vi "PicoScope4000ExampleStreaming.vi"() -> ()   [LabVIEW 2012]
doc: "This example demonstrates how to use the PicoScope Labview library to stream data from a PicoScope 4000 Series Device"
uses:
  PicoScope4000Lib/PicoScope4000AnalogChannelSettingsIEPE.ctl
  PicoScope4000Lib/PicoScope4000Buffer and Transfer Settings.ctl
panel:
  in  "Channel B Settings":T1={"Enabled"=FALSE, "Range"=6, "Bandwidth Limit"=0, "Coupling"=1} {"Coupling" items=["AC", "DC", "IEPE"]; "Bandwidth Limit" items=["Off", "200kHz"]; "Range" items=["10 mV", "20 mV", "50 mV", "100 mV", "200 mV", "500 mV", "1 V", "2 V", "5 V", "10 V", "20 V", "50 V ", "100 V"]}
  out "Unit Info":T2
  in  "Channel A Settings":T1={"Enabled"=TRUE, "Range"=6, "Bandwidth Limit"=0, "Coupling"=1} {"Coupling" items=["AC", "DC", "IEPE"]; "Bandwidth Limit" items=["Off", "200kHz"]; "Range" items=["10 mV", "20 mV", "50 mV", "100 mV", "200 mV", "500 mV", "1 V", "2 V", "5 V", "10 V", "20 V", "50 V ", "100 V"]}
  out "Analog Channels":cluster{i32, dbl, "Data (Volts)":dbl[]}[](graph)=[{0, 8e-09, "Data (Volts)"=[]}, {0, 8e-09, "Data (Volts)"=[]}, {0, 8e-09, "Data (Volts)"=[]}, {0, 8e-09, "Data (Volts)"=[]}, {0, 8e-09, "Data (Volts)"=[]}, {0, 8e-09, "Data (Volts)"=[]}, {0, 8e-09, "Data (Volts)"=[]}, {0, 8e-09, "Data (Volts)"=[]}]
  out "Raw Sample Interval (sec)":dbl format="%#.5p"
  out "Max ADC value":i16
  out "Chunk time(ms)":u32
  out "Elapsed time":dbl
  in  "Data file":path=path "PicoScope4000aExampleStreaming ChA Data"
  out "size(s)":i32
  out "Queue depth":i32(graph)
  out "queue depth":i32
  in  "Buffer and Transfer Settings":T3={"startIndex"=0, "Samples"=1000000, "Down Sample Ratio"=1, "Down-Sample Mode"=0} {"Down-Sample Mode" items=["None", "Aggregate", "Average"]; "Down Sample Ratio" step=1; "Samples" format="%_6p"}
  out "TriggeredAt (In Buffer)":u32 format="%#.6p"
  out "TriggeredAt (Total samples)":u32 format="%#.6p"
  in  "Acquisition Settings":T4={"Auto Stop"=TRUE, "Desired Sample Interval"=1, "Pre-trigger Samples"=0, "Post-trigger Samples"=1000000, "Down-Sample Ratio"=1, "Down-Sample Mode"=0, "Time Units"=3} {"Time Units" items=["Nanoseconds (ns)"=2, "Microseconds (us)"=3, "Milliseconds (ms)"=4, "Seconds (s)"=5]; "Down-Sample Mode" items=["None"=0, "Aggregate"=1, "Decimate"=2, "Average"=4]; "Post-trigger Samples" format="%#.6p"; "Pre-trigger Samples" format="%#_6p"}
  out "Triggered":bool
  out "DownSample Interval (sec)":dbl format="%#.5p"
  out "Total Samples":u32 format="%#.6p"
  out "Auto Stopped":bool
  in  "Serial Number":string
  in  "Open Using Serial Number":bool
  out "Number of Samples per Capture":u32 format="%#.6p"
  in  "Apply  Settings":bool
  in  "stop":bool
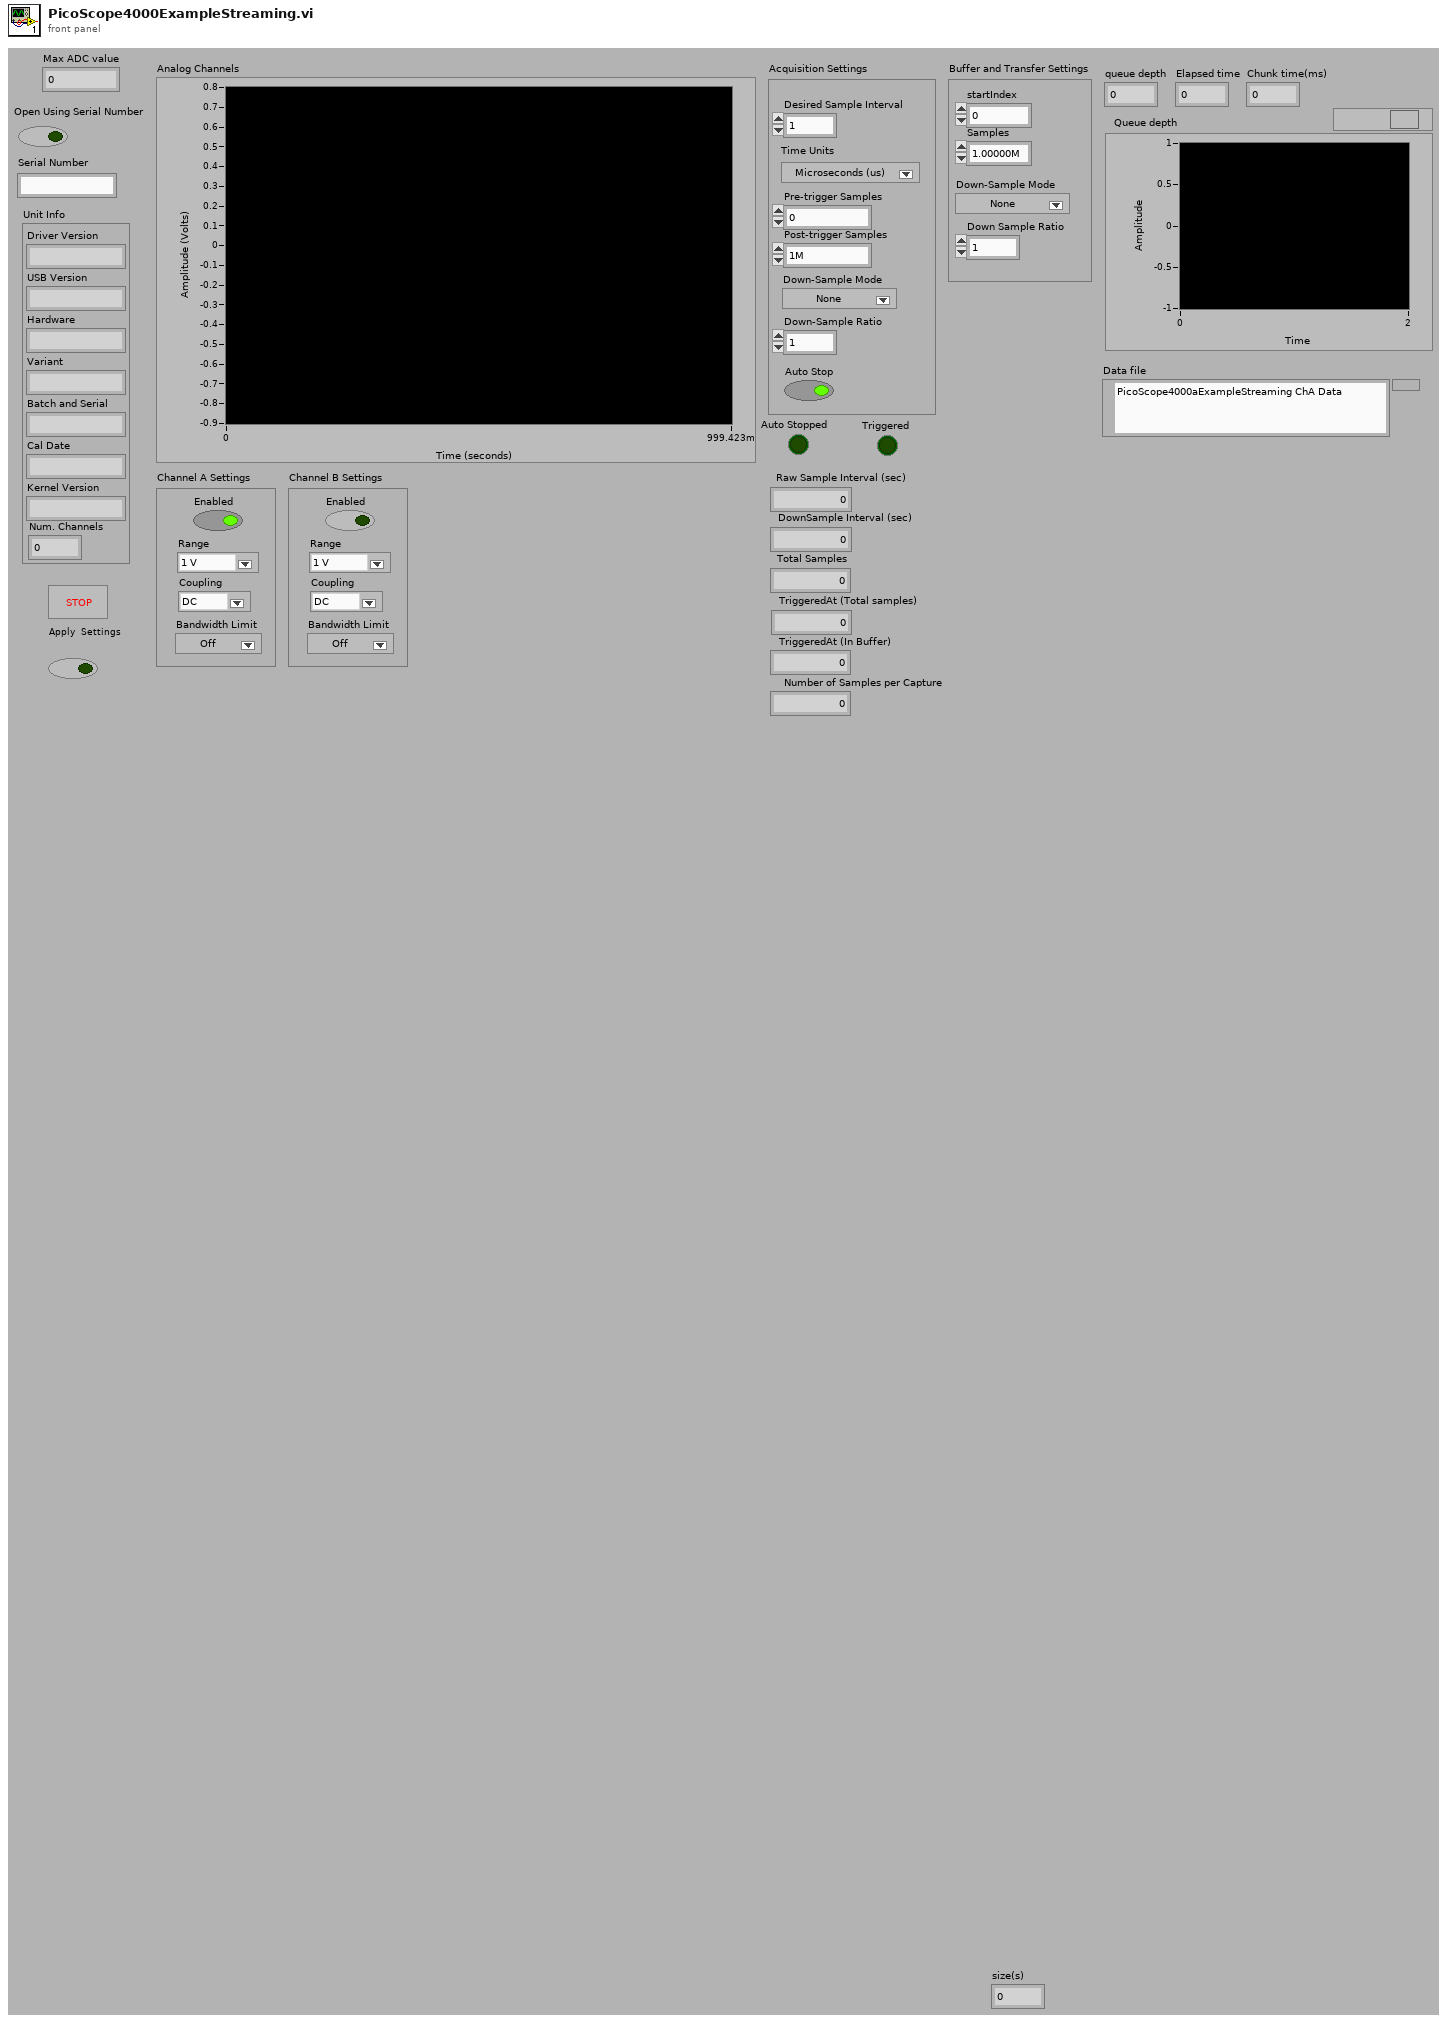
[diagram p1: front panel]
types:
  T1 = typedef "PicoScope4000AnalogChannelSettingsIEPE.ctl" = cluster{"Enabled":bool, "Range":u16, "Bandwidth Limit":i16, "Coupling":u16}
  T2 = cluster{"Driver Version":string, "USB Version":string, "Hardware":string, "Variant":string, "Batch and Serial":string, "Cal Date":string, "Kernel Version":string, "Num. Channels":i16}
  T3 = typedef "PicoScope4000Buffer and Transfer Settings.ctl" = cluster{"startIndex":u64, "Samples":u64, "Down Sample Ratio":u64, "Down-Sample Mode":u32}
  T4 = cluster{"Auto Stop":bool, "Desired Sample Interval":u32, "Pre-trigger Samples":u32, "Post-trigger Samples":u32, "Down-Sample Ratio":u32, "Down-Sample Mode":i32, "Time Units":u32}
  T5 = enum16{"open", "open or create", "create or replace", "create", "open (read-only)"}
  T6 = cluster{"Channel A Buffer":i16[], "Channel B Buffer":i16[], "Channel C Buffer":i16[], "Channel D Buffer":i16[], "Channel E Buffer":i16[], "Channel F Buffer":i16[], "Channel G Buffer":i16[], "Channel H Buffer":i16[], "Port 0":i16[], "Port 1":i16[]}
  T7 = cluster{i32, "DownSample Interval (sec)":dbl, "Data":dbl[]}
  T8 = cluster{i32, "DownSample Interval (sec)":dbl, "Data":dbl[]}[]
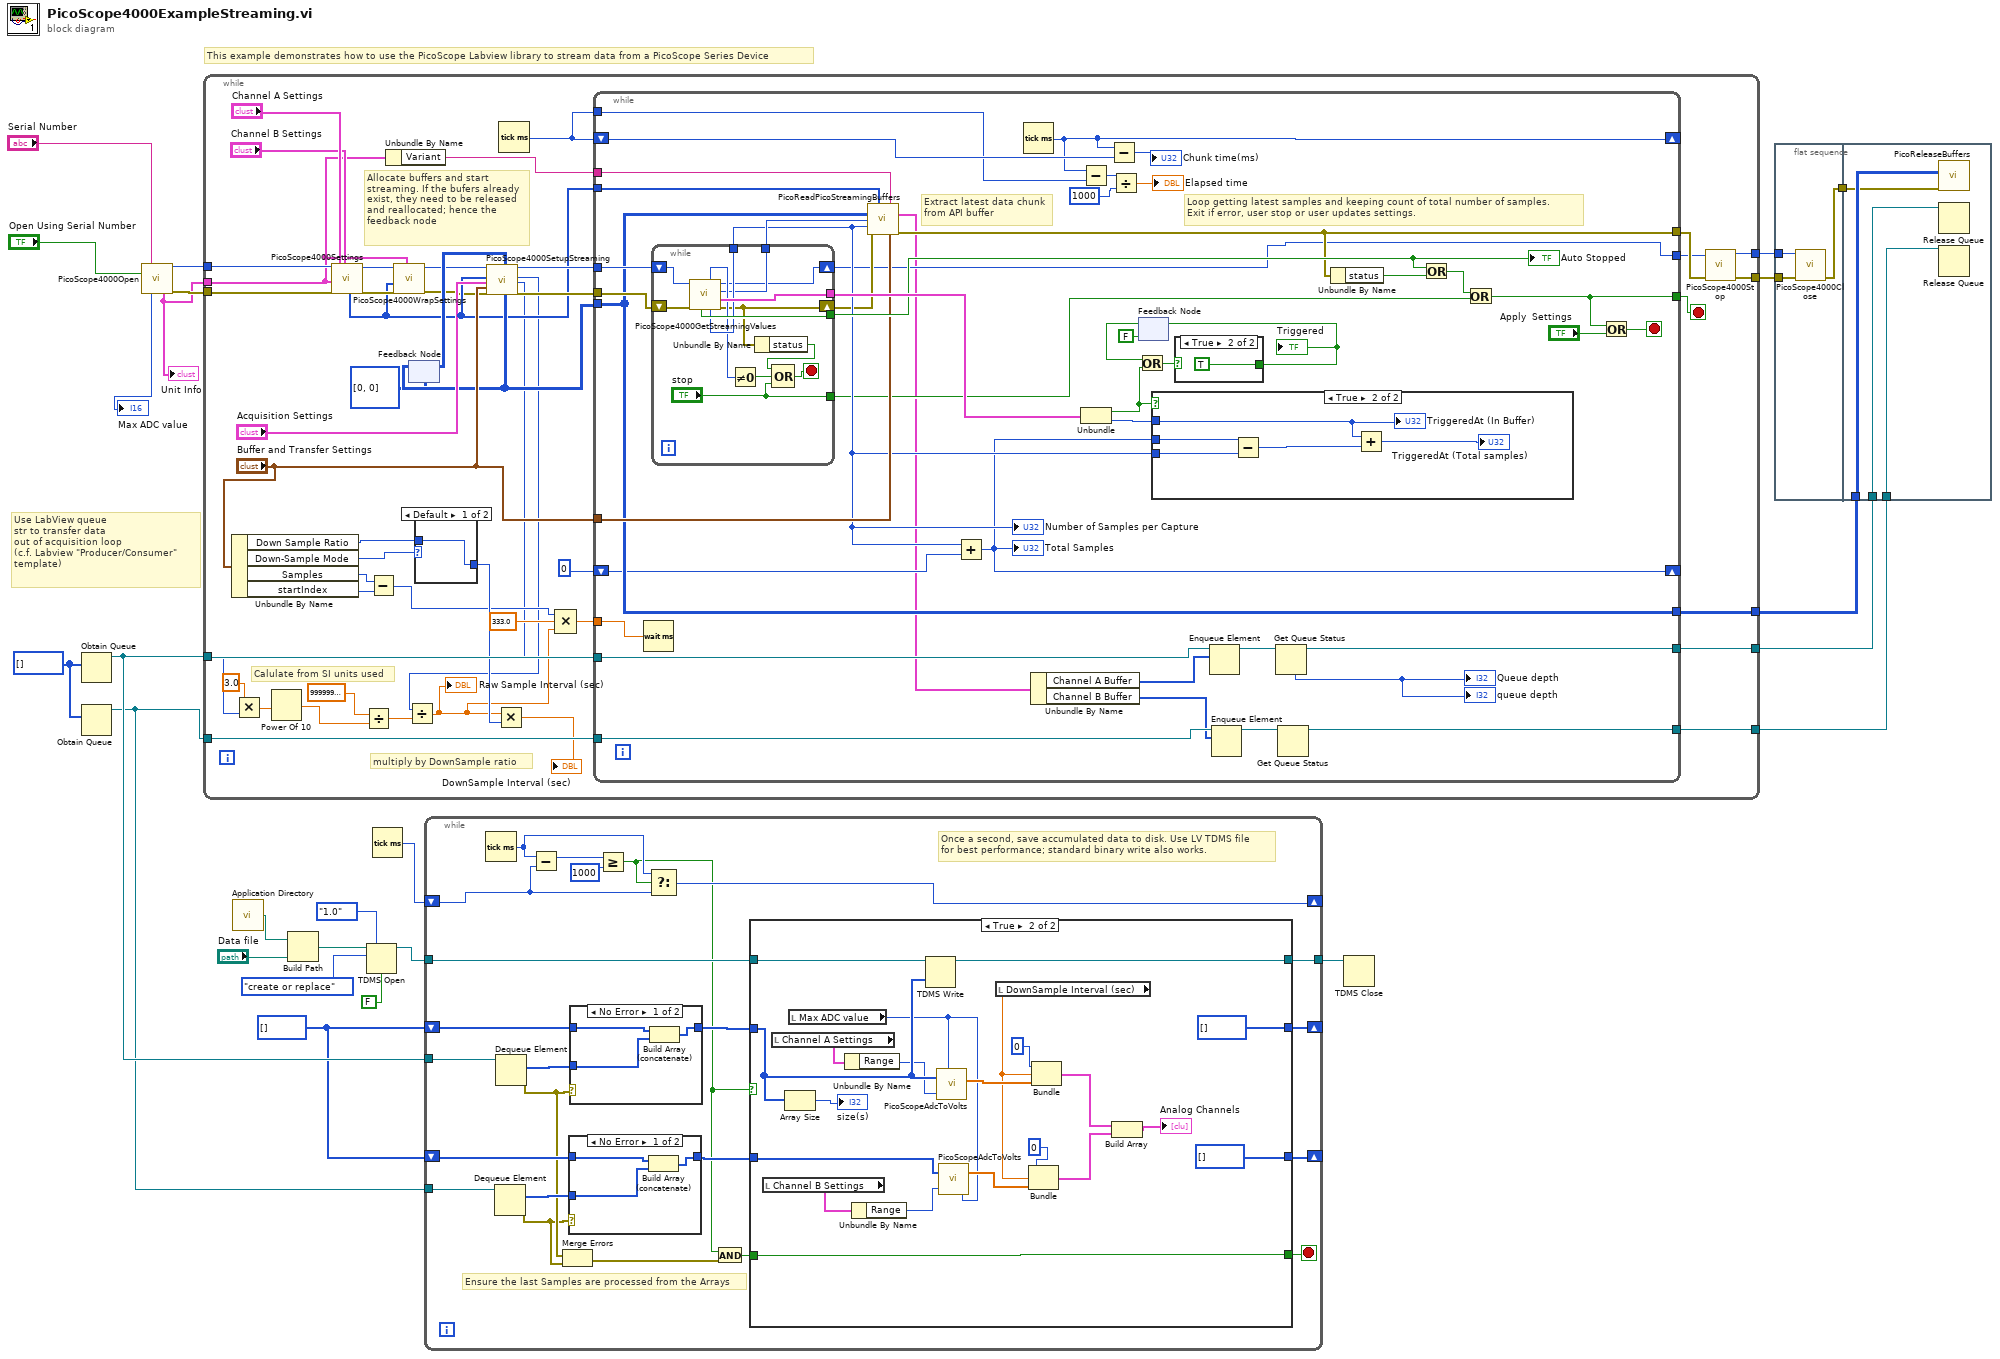
[diagram p0: block diagram]
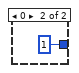
[diagram p5: hidden frame]
diagram:
  w12 = i16[] [] ("History Data")
  w15 = i16[] [] ("History Data")
  # "Use LabView queue\nstr to transfer data\nout of acquisition loop\n(c.f. Labview \"Producer/Consumer\"\ntemplate)"
  # "This example demonstrates how to use the PicoScope Labview library to stream data from a PicoScope Series Device"
  n1 = Obtain Queue(element data type=w15) -> (queue out=w25:refnum<queue>)  [unwired: 4 in, 2 out]
  n2 = Obtain Queue(element data type=w15) -> (queue out=w13:refnum<queue>)  [unwired: 4 in, 2 out]
  n3 = call "PicoScope4000Open.vi"("Serial Number"="Serial Number", "Use Serial Number"="Open Using Serial Number") -> ("handle"=w5:i16, "Max ADC value"=→"Max ADC value":i16, "Unit Info"=w3:T2, "error out"=w4:errorcluster)  [unwired: 10 in]
  "Unit Info" <- w3
  n4 = while {
    tunnel: [w57] -> w24
    tunnel: w5 -> [w71]
    tunnel: [w66] -> w22
    tunnel: w25 -> [w65]
    tunnel: [w37] -> w23
    tunnel: [w61] -> w14
    tunnel: w13 -> [w60]
    tunnel: w4 -> [w42]
    tunnel: w3 -> [w38]
    tunnel: [w26] -> w2
    stop <- w72 stop-if-true
    # "multiply by DownSample ratio"
    # "Calulate from SI units used"
    # "Allocate buffers and start\nstreaming. If the bufers already\nexist, they need to be released\nand reallocated; hence the\nfeedback node"
    n5 = Unbundle By Name("Buffer and Transfer Settings") -> ("Down Sample Ratio"=w69:u64, "Down-Sample Mode"=w70:u32, "Samples"=w48:u64, "startIndex"=w47:u64)
    n6 = call "PicoScope4000Settings.vi"("handle in"=w71, "Unit Info"=w38, "error in"=w42, "Channel A Settings"="Channel A Settings", "Channel B Settings"="Channel B Settings") -> ("Enabled array"=w30:i16[], "handle out"=w34:i16, "error out"=w35:errorcluster)  [unwired: 12 in]
    n7 = Subtract(x=w48, y=w47) -> (x-y=w46:u64)
    n8 = Unbundle By Name(w38) -> ("Variant"=w39:string)
    n9 = call "PicoScope4000WrapSettings.vi"("Unit Info"=w38, "error in (no error)"=w35, "Enabled array"=w30, "Handle In"=w34) -> ("error out"=w29:errorcluster, "Handle Out"=w33:i16)  [unwired: 6 in]
    n10 = feedback #1(u64[][] [[0], [0]] ("Pointer array")) -> (w64:u64[][])
    n11 = case shown="Default" w70 {
      tunnel: [w73 u32 1 ("Down-Sample Ratio")] -> w50
      tunnel: w69 -> [w73 _]
      frame Default {
      }
      frame 0 {
      }
    }
    n12 = call "PicoScope4000SetupStreaming.vi"("handle in"=w33, "enabled array"=w30, "Acquisition Settings"="Acquisition Settings", "Buffer and Transfer Settings"="Buffer and Transfer Settings", "error in"=w29, "Pointers In"=w64) -> ("Pointer array"=w63:u64[][], "handle out"=w32:i16, "Sample Interval"=w28:u32, "sampleIntervalTimeUnits"=w27:u32, "error out"=w31:errorcluster)  [unwired: 9 in]
    n13 = Multiply(x=3.0, y=w27) -> (x*y=w55:dbl)
    n14 = Power Of 10(x=w55) -> (10^x=w54:dbl)
    n15 = Divide(x=sgl 1000000000000000.0 ("y"), y=w54) -> (x/y=w51:dbl)
    n16 = Divide(x=w28, y=w51) -> (x/y=w43:dbl)
    "Raw Sample Interval (sec)" <- w43
    n17 = feedback-in #1(w63) -> ()
    n18 = Multiply(x=w43, y=w50) -> (x*y=→"DownSample Interval (sec)":dbl)
    n19 = Tick Count (ms)() -> (millisecond timer value=w56:u32)
    n20 = Compound Arithmetic op=MULTIPLY(w46, 333.0 ("value"), w43) -> (w49:dbl)
    n21 = while {
      tunnel: [w76] -> w58
      tunnel: [w118] -> w72
      tunnel: w31 -> [w106]
      tunnel: w32 -> [w105]
      tunnel: [w103] -> w59
      tunnel: "Buffer and Transfer Settings" -> [w104]
      tunnel: w30 -> [w102]
      tunnel: [w100] -> w66
      tunnel: w65 -> [w98]
      tunnel: w63 -> [w97]
      tunnel: [w97] -> w37
      shift-right: [w92] -> _
      shift-left: w56 -> [w93]
      tunnel: w39 -> [w87]
      tunnel: [w85] -> w61
      tunnel: w60 -> [w84]
      tunnel: w56 -> [w81]
      tunnel: w49 -> [w80]
      shift-right: [w78] -> _
      shift-left: u32 0 -> [w79]
      stop <- w117 stop-if-true
      # "Loop getting latest samples and keeping count of total number of samples. \nExit if error, user stop or user updates settings."
      # "Extract latest data chunk\nfrom API buffer"
      n22 = Wait (ms)(milliseconds to wait=w80) -> ()  [unwired: 1 out]
      n23 = while {
        tunnel: [w132] -> w116
        tunnel: [w131] -> w113
        tunnel: [w124] -> w89
        tunnel: [w130] -> w88
        shift-right: [w120] -> w77
        shift-left: w106 -> [w121]
        shift-right: [w122] -> w76
        shift-left: w105 -> [w123]
        tunnel: ["stop"] -> w82
        stop <- w126 stop-if-true
        n24 = call "PicoScope4000GetStreamingValues.vi"("error in"=w121, "handle in"=w123) -> ("error out"=w120:errorcluster, "Trigger"=w132:cluster{bool, "triggeredAt (Total samples)":u32}, "Start Index in Driver Buffer"=w124:u32, "handle out"=w122:i16, "Number of Samples"=w130:u32, "ready"=w129:i16, "Auto Stopped"=w131:bool)  [unwired: 3 in]
        n25 = Not Equal To 0?(x=w129) -> (x != 0?=w127:bool)
        n26 = Unbundle By Name(w120) -> ("status"=w128:bool)
        n27 = Compound Arithmetic op=OR(w128, w127, "stop") -> (w126:bool)
      }
      "Number of Samples per Capture" <- w88
      "Auto Stopped" <- w113
      n28 = call "PicoReadPicoStreamingBuffers.vi"("enabled array"=w102, "Buffer and Transfer Settings"=w104, "Variant"=w87, "Pointer array"=w97, "Offset Index"=w89, "Number of Samples"=w88, "error in (no error)"=w77) -> ("Buffers (Max or non-aggregated)"=w75:T6, "error out"=w103:errorcluster)  [unwired: 6 in, 1 out]
      n29 = Add(x=w88, y=w79) -> (x+y=w78:u32)
      "Total Samples" <- w78
      n30 = Tick Count (ms)() -> (millisecond timer value=w92:u32)
      n31 = Unbundle By Name(w75) -> ("Channel A Buffer"=w90:i16[], "Channel B Buffer"=w83:i16[])
      n32 = Subtract(x=w92, y=w81) -> (x-y=w96:u32)
      n33 = Unbundle(w116) -> (w108:bool, "triggeredAt (Total samples)"=w107:u32)
      n34 = Subtract(x=w92, y=w93) -> (x-y=→"Chunk time(ms)":u32)
      n35 = Divide(x=w96, y=u32 1000) -> (x/y=→"Elapsed time":dbl)
      n36 = feedback #2(FALSE) -> (w112:bool)
      n37 = Or(x=w112, y=w108) -> (x .or. y?=w110:bool)
      n38 = case shown="True" w108 {
        tunnel: w88 -> [_ w133]
        tunnel: w78 -> [_ w137]
        tunnel: w107 -> [_ w135]
        frame False {
        }
        frame True {
          n39 = Subtract(x=w137, y=w133) -> (x-y=w136:u32)
          n40 = Add(x=w135, y=w136) -> (x+y=→"TriggeredAt (Total samples)":u32)
          "TriggeredAt (In Buffer)" <- w135
        }
      }
      n41 = case shown="True" w110 {
        selector: w110 -> [w138 _]
        tunnel: [w138 TRUE] -> w109
        frame False {
        }
        frame True {
        }
      }
      "Triggered" <- w109
      n42 = feedback-in #2(w109) -> ()
      n43 = Enqueue Element(queue=w98, element=w90) -> (queue out=w99:refnum<queue>)  [unwired: 2 in, 2 out]
      n44 = Enqueue Element(queue=w84, element=w83) -> (queue out=w86:refnum<queue>)  [unwired: 2 in, 2 out]
      n45 = Get Queue Status(queue=w99) -> (queue out=w100:refnum<queue>, # elements in queue=→"queue depth" →"Queue depth":i32)  [unwired: 2 in, 6 out]
      n46 = Get Queue Status(queue=w86) -> (queue out=w85:refnum<queue>)  [unwired: 2 in, 7 out]
      n47 = Unbundle By Name(w103) -> ("status"=w115:bool)
      n48 = Or(x=w113, y=w115) -> (x .or. y?=w114:bool)
      n49 = Or(x=w114, y=w82) -> (x .or. y?=w118:bool)
      n50 = Or(x=w118, y="Apply  Settings") -> (x .or. y?=w117:bool)
    }
    n51 = call "PicoScope4000Stop.vi"("error in (no error)"=w59, "handle in"=w58) -> ("error out"=w26:errorcluster, "handle out"=w57:i16)  [unwired: 8 in]
  }
  n52 = call <vilib>:"Application Directory.vi"() -> ("Application Directory"=w9:path)
  n53 = Build Path(base path=w9, name or relative path="Data file") -> (appended path=w10:path)
  n54 = TDMS Open(6:FALSE ("disable buffering? (T)"), 7:enum16{"1.0", "2.0"}."1.0" ("file format version (2.0)"), 10:T5."create or replace" ("operation (0:open)"), 11:w10) -> (3:w19:refnum<k34>)  [unwired: 2 in, 1 out]
  n55 = Tick Count (ms)() -> (millisecond timer value=w21:u32)
  n56 = while {
    tunnel: w25 -> [w161]
    shift-right: [w153] -> _
    shift-left: w12 -> [w160]
    shift-right: [w155] -> _
    shift-left: w21 -> [w156]
    tunnel: w19 -> [w152]
    tunnel: [w151] -> w18
    tunnel: w13 -> [w149]
    shift-right: [w146] -> _
    shift-left: w12 -> [w148]
    stop <- w143 stop-if-true
    # "Ensure the last Samples are processed from the Arrays"
    # "Once a second, save accumulated data to disk. Use LV TDMS file\nfor best performance; standard binary write also works."
    n57 = Tick Count (ms)() -> (millisecond timer value=w157:u32)
    n58 = Dequeue Element(queue=w149) -> (element=w150:i16[], error out=w144:errorcluster)  [unwired: 2 in, 2 out]
    n59 = Dequeue Element(queue=w161) -> (element=w162:i16[], error out=w145:errorcluster)  [unwired: 2 in, 2 out]
    n60 = Subtract(x=w157, y=w156) -> (x-y=w159:u32)
    n61 = Merge Errors(w145, w144) -> (w142:errorcluster)
    n62 = case shown="No Error" w144 {
      tunnel: w148 -> [w165 w166]
      tunnel: [w164 w166] -> w147
      tunnel: w150 -> [w163 _]
      frame No Error {
        n63 = Build Array (concatenate)(w165, w163) -> (w164:i16[])
      }
      frame Error {
      }
    }
    n64 = case shown="No Error" w145 {
      tunnel: w160 -> [w194 w195]
      tunnel: [w193 w195] -> w154
      tunnel: w162 -> [w192 _]
      frame No Error {
        n65 = Build Array (concatenate)(w194, w192) -> (w193:i16[])
      }
      frame Error {
      }
    }
    n66 = Greater Or Equal?(x=w159, y=u32 1000) -> (x >= y?=w141:bool)
    n67 = Select(t=w157, s=w141, f=w156) -> (s? t:f=w155:u32)
    n68 = And(x=w141, y=w142) -> (x .and. y?=w140:bool)
    n69 = case shown="True" w141 {
      tunnel: w154 -> [w170 w187]
      tunnel: [w170 i16[] [] ("History Data")] -> w153
      tunnel: w152 -> [w169 w189]
      tunnel: [w169 w188] -> w151
      tunnel: w147 -> [w168 w175]
      tunnel: [w168 i16[] [] ("History Data")] -> w146
      tunnel: [w167 w173] -> w143
      tunnel: w140 -> [w167 w173]
      frame False {
      }
      frame True {
        n70 = local read "Channel B Settings"() -> (w171:T1)
        n71 = local read "Channel A Settings"() -> (w172:T1)
        n72 = Array Size(array=w187) -> (size(s)=→"size(s)":i32)
        n73 = local read "Max ADC value"() -> (w177:i16)
        n74 = Unbundle By Name(w172) -> ("Range"=w186:u16)
        n75 = Unbundle By Name(w171) -> ("Range"=w176:u16)
        n76 = TDMS Write(0:w189, 9:w187) -> (4:w188:refnum<k34>)  [unwired: 4 in, 3 out]
        n77 = call "PicoScopeAdcToVolts.vi"("Max_adc"=w177, "Range Index"=w186, "Data"=w187) -> ("Data"=w184:dbl[])
        n78 = call "PicoScopeAdcToVolts.vi"("Max_adc"=w177, "Range Index"=w176, "Data"=w175) -> ("Data"=w182:dbl[])
        n79 = local read "DownSample Interval (sec)"() -> (w181:dbl)
        n80 = Bundle(0, "DownSample Interval (sec)"=w181, "Data"=w182) -> (w178:T7)  [unwired: 1 in]
        n81 = Bundle(0, "DownSample Interval (sec)"=w181, "Data"=w184) -> (w179:T7)  [unwired: 1 in]
        n82 = Build Array(w179, w178) -> (→"Analog Channels":T8)
      }
    }
  }
  n83 = TDMS Close(11:w18) -> ()  [unwired: 1 in, 2 out]
  n84 = flat-sequence {
    tunnel: w24 -> [w198]
    tunnel: w2 -> [w197]
    tunnel: [w196] -> w1
    tunnel: w23 -> [w202]
    tunnel: w22 -> [w201]
    tunnel: w14 -> [w200]
    tunnel: w1 -> [w199]
    frame #0 {
      n85 = call "PicoScope4000Close.vi"("error in (no error)"=w197, "handle"=w198) -> ("error out"=w196:errorcluster)  [unwired: 9 in]
    }
    frame #1 {
      n86 = call "PicoReleaseBuffers.vi"("error in (no error)"=w199, "Pointer array"=w202) -> ()  [unwired: 9 in, 1 out]
      n87 = Release Queue(queue=w201) -> ()  [unwired: 2 in, 3 out]
      n88 = Release Queue(queue=w200) -> ()  [unwired: 2 in, 3 out]
    }
  }
